vi "ncs_breath.vi"() -> ()   [LabVIEW 2016]
uses:
  <instrlib>/niUSRP/niUSRP Timestamp.ctl
  <instrlib>/niUSRP/niUSRP Write Tx Data (2D CDB).vi
  <instrlib>/niUSRP/niUSRP Fetch Rx Data (2D CDB).vi
  <vilib>/measure/maspectr.llb/FFT Power Spectrum for 1 Chan (CDB).vi
  <vilib>/Analysis/NI_AALBase.lvlib
  <vilib>/Analysis/3filter.llb/Filter Passband Type.ctl
  <vilib>/Analysis/baseanly.llb/IIR Cascade Filter (DBL).vi
  <vilib>/measure/NI_MAPro.lvlib
panel:
  out "Rx Channel tone":dbl
  in  "Preset":string="v1a"
  out "Alarm":bool
  in  "Epsilon":dbl=0.05 format="%#_13g"
  in  "Timer":u16(ring)=90 items=["20min"=1200, "11min"=660, "10min"=600, "5.5min"=330, "2.5min"=150, "1.5min"=90]
  out "Elapsed Time (s)":dbl
  out "Time has Elapsed":bool
  in  "Timer Start":bool
  in  "File Name":string="freq2G_1"
  in  "Path":path=path "D:/Research/SummerFall17Spring18/CnC/NCS/Respiratory/BreathPattern_Cough_Speak/Data"
  out "NCS heartbeat":dbl[](graph)
  in  "Order":dbl=20.0 format="%#_13g"
  in  "High-Cutoff":dbl=8.0 format="%#_13g"
  in  "Low-Cutoff":dbl=0.5 format="%#_13g"
  out "size(s)":i32
  out "Coerced Rx IQ Rate":dbl
  in  "Sampling Rate":i32=500
  out "Gain":dbl=-15.0
  out "Bandwidth":dbl=56000000.0
  out "Coerced Carrier Freq":dbl=2000000000.0 format="%#.17g"
  out "Coerced Tx IQ rate":dbl=1000000.0
  out "error IO":errorcluster={"status"=FALSE, "code"=-1074118647, "source"=""}
  in  "Rx #Samples":i32=20000
  in  "Tab Control 2":enum32{"NI-294x/295x", "NI-2900/2901"}(tab)=enum."NI-2900/2901"
  in  "Rx carrier frequency [Hz]":dbl=2000000000.0 format="%#_6p"
  in  "Tx carrier frequency [Hz]":dbl=1000000000.0 format="%#_6p"
  in  "Start Trigger Time":T1={"whole seconds"=1, "fractional seconds"=0.0}
  in  "Tab Control":T2(tab)
  out "NCS tag Amp":dbl[](graph)=[0.011967714738528729, 0.012021355192189592, 0.012015275039596582, 0.011969166030167903, 0.011958890166168242, 0.012007893820858737, 0.012022893722444085, 0.011978222225113794, 0.011969989939463181, 0.012003099640895068]
  out "NCS tag Phase":dbl[](graph)=[0.011967714738528729, 0.012021355192189592, 0.012015275039596582, 0.011969166030167903, 0.011958890166168242, 0.012007893820858737, 0.012022893722444085, 0.011978222225113794, 0.011969989939463181, 0.012003099640895068]
  out "Tag Amp":dbl[](graph)
  out "Tag Phase":dbl[](graph)
  out "Tx Waveform Graph":waveform(dbl)[](graph)
  out "Baseband Power Spectrum":cluster{"f0":dbl, "df":dbl, "magnitude":dbl[]}[](graph)
  in  "Stop":bool
  in  "Tone Amplitude":dbl=0.707 step=0.05 format="%#.6g"
  in  "Tone Frequency":dbl=10000.0 format="%#_6p"
  in  "Tx Waveform Size":dbl=200.0
  in  "Device Name":refnum<k15>="MyB210"
  in  "Tx Gain":dbl=28.0 format="%#_6f"
  in  "Tx IQ Rate":dbl=1000000.0 format="%#_6p"
  in  "Rx Gain":dbl=32.0 format="%#_6f"
  in  "Rx IQ Rate":dbl=250000.0 format="%#_6p"
  # "Note that on the NI-2900 and NI-2901, both Rx channels share an LO and both Tx channels share an LO. However, on the NI-294x/295x devices, Rx and Tx of channel 0 share an LO and Rx and Tx of channel 1 share an LO."
  # "Rx Settings"
  # "Tx Settings"
  # "Channel 0"
  # "Heartbeat Filter"
  # "This Tx graph should always have end and start tied up since this is being sent in a loop continuously. Otherwise phase jumps will be noticed."
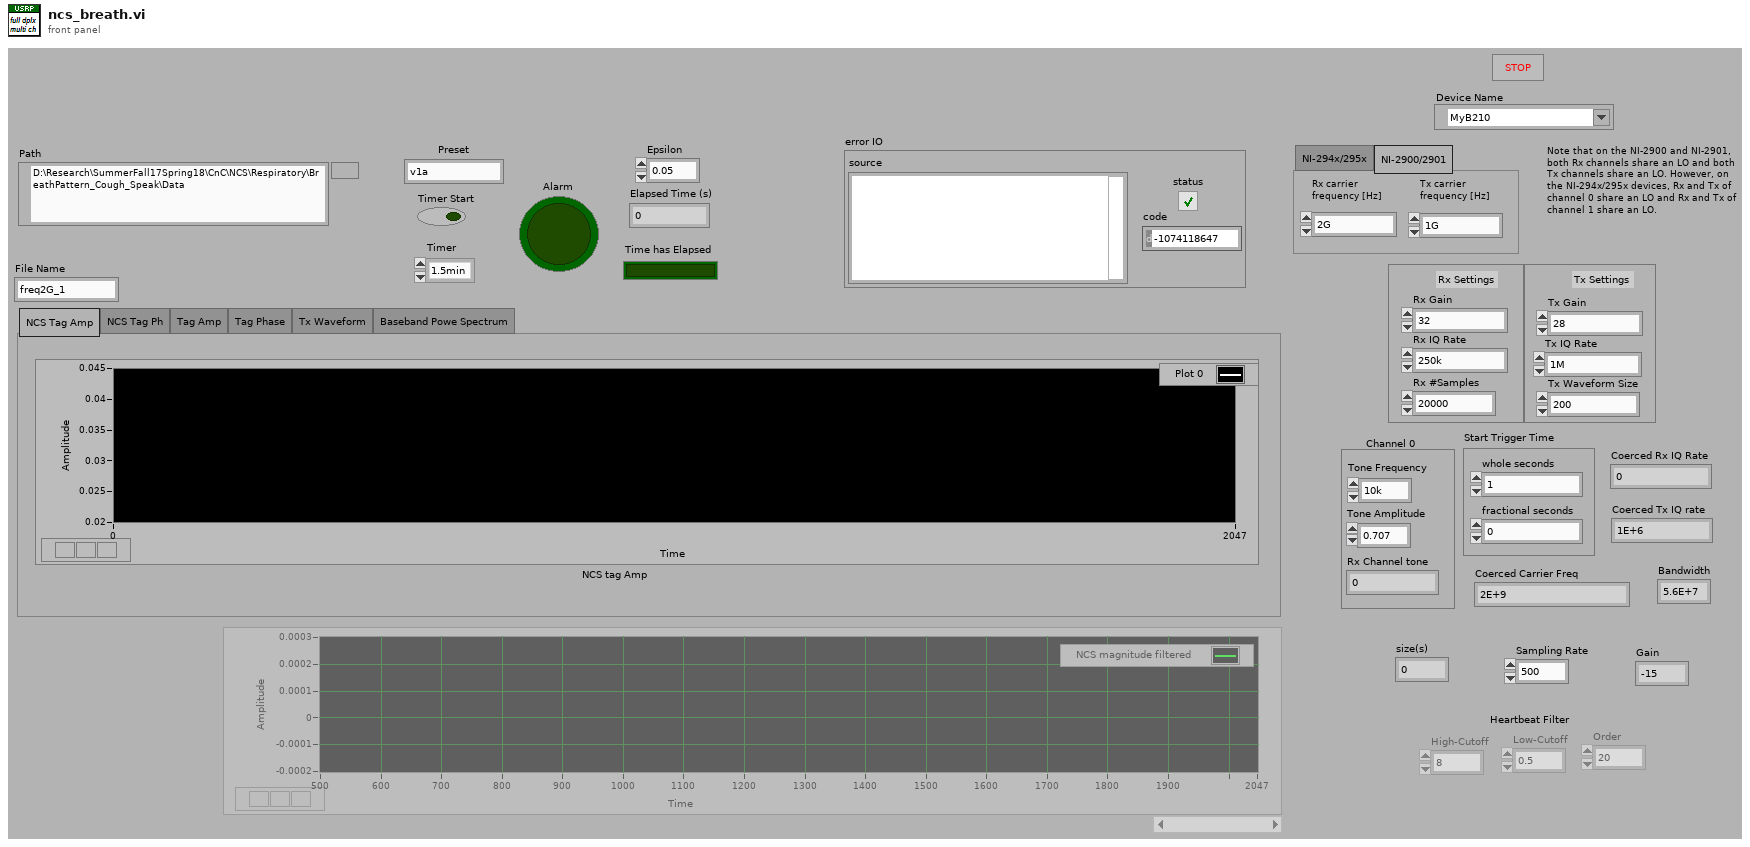
[diagram p1: front panel]
types:
  T1 = typedef "niUSRP Timestamp.ctl" = cluster{"whole seconds":u64, "fractional seconds":dbl}
  T2 = enum32{"NCS Tag Amp", "NCS Tag Ph", "Tag Amp", "Tag Phase", "Tx Waveform", "Baseband Powe Spectrum"}
  T3 = typedef "NI_AALBase.lvlib/Filter Passband Type.ctl" = enum32{"Lowpass", "Highpass", "Bandpass", "Bandstop"}
  T4 = cluster{"filter structure":enum32{"IIR 2nd Order", "IIR 4th Order"}, "Reverse Coefficients":dbl[], "Forward Coefficients":dbl[]}
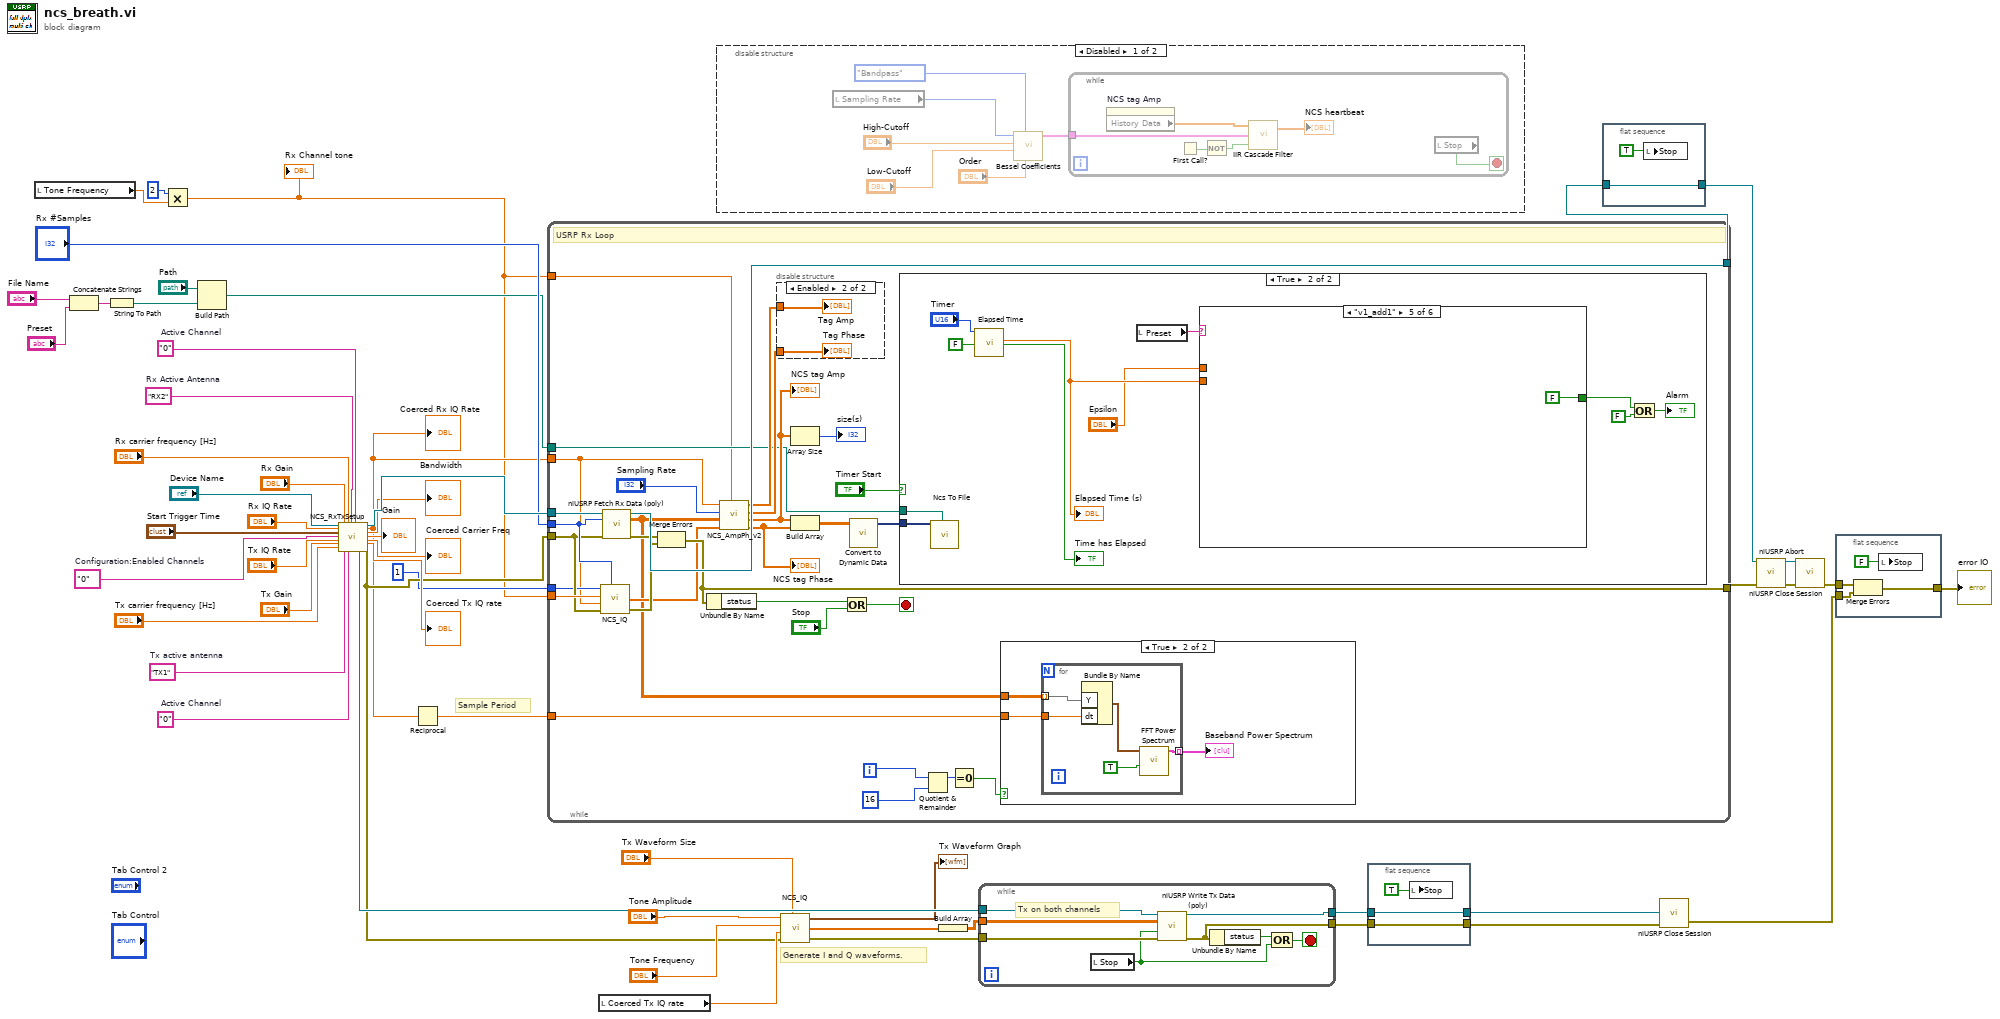
[diagram p0: block diagram]
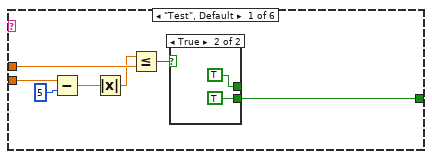
[diagram p5: hidden frame]
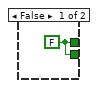
[diagram p6: hidden frame]
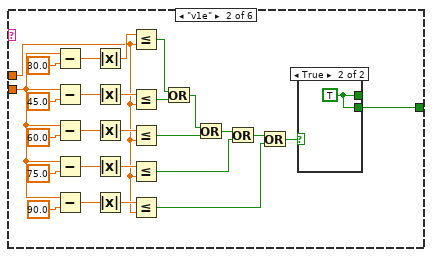
[diagram p7: hidden frame]
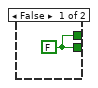
[diagram p8: hidden frame]
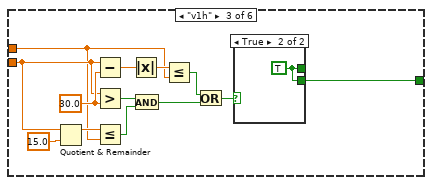
[diagram p9: hidden frame]
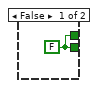
[diagram p10: hidden frame]
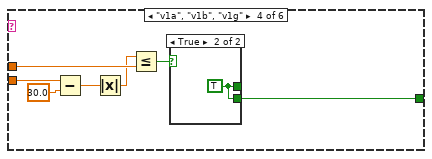
[diagram p11: hidden frame]
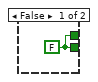
[diagram p12: hidden frame]
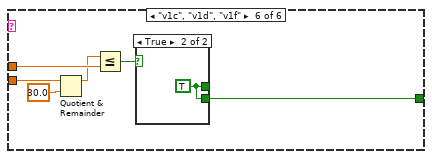
[diagram p13: hidden frame]
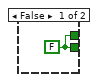
[diagram p14: hidden frame]
diagram:
  w10 = "0"  # Active Channel
  w11 = "0"  # Active Channel
  w45 = "RX2"  # Rx Active Antenna
  w41 = "TX1"  # Tx active antenna
  w27 = "0"  # Configuration:Enabled Channels
  # "Sample Period"
  # "Generate I and Q waveforms."
  n1 = local read "Tone Frequency"() -> (w26:dbl)
  n2 = Concatenate Strings("File Name", "Preset") -> (w5:string)
  n3 = String To Path(string=w5) -> (path=w9:path)
  n4 = Multiply(x=2, y=w26) -> (x*y=w1:dbl)
  "Rx Channel tone" <- w1
  n5 = Build Path(base path="Path", name or relative path=w9) -> (appended path=w7:path)
  n6 = call "NCS_RxTxSetup.vi"("Device Name"="Device Name", "Rx IQ Rate"="Rx IQ Rate", "Start Trigger Time"="Start Trigger Time", "Configuration:Enabled Channels"=w27, "Tx IQ Rate"="Tx IQ Rate", "Tx Gain"="Tx Gain", "Tx carrier frequency [Hz]"="Tx carrier frequency [Hz]", "Rx Gain"="Rx Gain", "Tx active antenna"=w41, "Rx carrier frequency [Hz]"="Rx carrier frequency [Hz]", "Active Channel"=w10, "Rx Active Antenna"=w45, "Active Channel 2"=w11) -> ("Tx session handle out"=w52:refnum<k15>, "Rx Session Handle out"=w53:refnum<k15>, "Coerced Rx IQ Rate"=w3:dbl, "Bandwidth"=→"Bandwidth":dbl, "Gain"=→"Gain":dbl, "Carrier Frequency"=→"Coerced Carrier Freq":dbl, "IQ Rate 2"=→"Coerced Tx IQ rate":dbl, "error out"=w21:errorcluster)  [unwired: 7 in]
  "Coerced Rx IQ Rate" <- w3
  n7 = Reciprocal(x=w3) -> (1/x=w2:dbl)
  n8 = while {
    tunnel: w53 -> [w84]
    tunnel: w21 -> [w76]
    tunnel: [w83] -> w37
    tunnel: "Rx #Samples" -> [w78]
    tunnel: w3 -> [w72]
    tunnel: [w73] -> w29
    tunnel: w1 -> [w77]
    tunnel: 1 -> [w74]
    tunnel: w7 -> [w63]
    tunnel: w2 -> [w57]
    tunnel: w1 -> [w54]
    i -> [w56]
    stop <- w79 stop-if-true
    # "USRP Rx Loop"
    n9 = call "NCS_IQ.vi"("Tone Amplitude"=w74, "Waveform Size"=w78, "Tone Frequency"=w77, "Coerced IQ rate"=w72, "error in (no error)"=w76) -> ("IQ waveform array"=w71:cdb[], "error out"=w75:errorcluster)  [unwired: 1 in, 1 out]
    n10 = call-poly <instrlib>:"niUSRP Fetch Rx Data (poly).vi"("session handle"=w84, "number of samples"=w78, "error in (no error)"=w76) -> ("session handle out"=w83:refnum<k15>, "data"=w58:cdb[][], "error out"=w80:errorcluster)  [unwired: 9 in, 1 out]
    n11 = Merge Errors(w80, w75) -> (w73:errorcluster)
    n12 = Unbundle By Name(w73) -> ("status"=w82:bool)
    n13 = call "NCS_AmpPh_v2.vi"("Rx Channel Tone"=w54, "IQ"=w71, "data"=w58, "Sampling Rate"="Sampling Rate", "Coerced Rx IQ Rate"=w72) -> ("Phase DownSampled"=w64:dbl[], "Amp DownSampled"=w65:dbl[], "Phase"=w70:dbl[], "Amplitude"=w68:dbl[])  [unwired: 3 in]
    "NCS tag Amp" <- w65
    "NCS tag Phase" <- w64
    n14 = disable-structure shown="Enabled" {
      disable-tunnel: w68 -> [_ w177]
      disable-tunnel: w70 -> [_ w176]
      frame Disabled {
      }
      frame Enabled {
        "Tag Amp" <- w177
        "Tag Phase" <- w176
      }
    }
    n15 = Array Size(array=w65) -> (size(s)=→"size(s)":i32)
    n16 = Build Array(w65, w64) -> (w66:dbl[][])
    n17 = Or(x=w82, y="Stop") -> (x .or. y?=w79:bool)
    n18 = call "Convert to Dynamic Data"("2D Array"=w66) -> ("Dynamic Data Type"=w62:dynamicdata)  [unwired: 3 in]
    n19 = case shown="True" "Timer Start" {
      tunnel: w63 -> [_ w103]
      tunnel: w62 -> [_ w102]
      frame False {
      }
      frame True {
        n20 = call "Ncs To File"("Signals"=w102, "Filename"=w103) -> ()  [unwired: 15 in, 3 out]
        n21 = call "Elapsed Time"("Time Target (s)"="Timer", "Auto Reset"=FALSE) -> ("Elapsed Time (s)"=w98:dbl, "Time has Elapsed"=→"Time has Elapsed":bool)  [unwired: 10 in, 6 out]
        "Elapsed Time (s)" <- w98
        n22 = local read "Preset"() -> (w93:string)
        n23 = case shown="\"v1_add1\"" w93 {
          tunnel: w98 -> [w110 w121 w149 w162 _ w171]
          tunnel: "Epsilon" -> [w107 w115 w146 w161 _ w170]
          tunnel: [w106 w129 w152 w163 FALSE w172] -> w95
          frame "Test", Default {
            n24 = Subtract(x=w110, y=5) -> (x-y=w108:dbl)
            n25 = Absolute Value(x=w108) -> (abs(x)=w105:dbl)
            n26 = Less Or Equal?(x=w105, y=w107) -> (x <= y?=w104:bool)
            n27 = case shown="True" w104 {
              tunnel: [w111 TRUE] -> w106
              tunnel: [w111 TRUE] -> _
              frame False {
                w111 = FALSE
              }
              frame True {
              }
            }
          }
          frame "v1e" {
            n28 = Subtract(x=w121, y=30.0) -> (x-y=w139:dbl)
            n29 = Subtract(x=w121, y=45.0) -> (x-y=w136:dbl)
            n30 = Subtract(x=w121, y=60.0) -> (x-y=w132:dbl)
            n31 = Subtract(x=w121, y=75.0) -> (x-y=w128:dbl)
            n32 = Subtract(x=w121, y=90.0) -> (x-y=w124:dbl)
            n33 = Absolute Value(x=w139) -> (abs(x)=w138:dbl)
            n34 = Absolute Value(x=w136) -> (abs(x)=w135:dbl)
            n35 = Absolute Value(x=w132) -> (abs(x)=w131:dbl)
            n36 = Absolute Value(x=w128) -> (abs(x)=w127:dbl)
            n37 = Absolute Value(x=w124) -> (abs(x)=w123:dbl)
            n38 = Less Or Equal?(x=w138, y=w115) -> (x <= y?=w137:bool)
            n39 = Less Or Equal?(x=w135, y=w115) -> (x <= y?=w133:bool)
            n40 = Less Or Equal?(x=w131, y=w115) -> (x <= y?=w120:bool)
            n41 = Less Or Equal?(x=w127, y=w115) -> (x <= y?=w118:bool)
            n42 = Less Or Equal?(x=w123, y=w115) -> (x <= y?=w116:bool)
            n43 = Or(x=w137, y=w133) -> (x .or. y?=w125:bool)
            n44 = Or(x=w125, y=w120) -> (x .or. y?=w119:bool)
            n45 = Or(x=w119, y=w118) -> (x .or. y?=w117:bool)
            n46 = Or(x=w117, y=w116) -> (x .or. y?=w114:bool)
            n47 = case shown="True" w114 {
              tunnel: [w141 w142] -> _
              tunnel: [w141 w142] -> w129
              frame False {
                w141 = FALSE
              }
              frame True {
                w142 = TRUE
              }
            }
          }
          frame "v1h" {
            w151 = 30.0 ("y")
            n48 = Quotient & Remainder(x=w149, y=15.0) -> (x-y*floor(x/y)=w147:dbl)  [unwired: 1 out]
            n49 = Subtract(x=w149, y=w151) -> (x-y=w155:dbl)
            n50 = Greater?(x=w149, y=w151) -> (0:w150:bool)
            n51 = Less Or Equal?(x=w147, y=w146) -> (x <= y?=w145:bool)
            n52 = Absolute Value(x=w155) -> (abs(x)=w154:dbl)
            n53 = And(x=w150, y=w145) -> (x .and. y?=w144:bool)
            n54 = Less Or Equal?(x=w154, y=w146) -> (x <= y?=w153:bool)
            n55 = Or(x=w153, y=w144) -> (x .or. y?=w143:bool)
            n56 = case shown="True" w143 {
              tunnel: [w156 w157] -> _
              tunnel: [w156 w157] -> w152
              frame False {
                w156 = FALSE
              }
              frame True {
                w157 = TRUE
              }
            }
          }
          frame "v1a", "v1b", "v1g" {
            n57 = Subtract(x=w162, y=30.0) -> (x-y=w159:dbl)
            n58 = Absolute Value(x=w159) -> (abs(x)=w158:dbl)
            n59 = Less Or Equal?(x=w158, y=w161) -> (x <= y?=w160:bool)
            n60 = case shown="True" w160 {
              tunnel: [w165 w166] -> _
              tunnel: [w165 w166] -> w163
              frame False {
                w165 = FALSE
              }
              frame True {
                w166 = TRUE
              }
            }
          }
          frame "v1_add1" {
          }
          frame "v1c", "v1d", "v1f" {
            n61 = Quotient & Remainder(x=w171, y=30.0) -> (x-y*floor(x/y)=w168:dbl)  [unwired: 1 out]
            n62 = Less Or Equal?(x=w168, y=w170) -> (x <= y?=w169:bool)
            n63 = case shown="True" w169 {
              tunnel: [w174 w175] -> _
              tunnel: [w174 w175] -> w172
              frame False {
                w174 = FALSE
              }
              frame True {
                w175 = TRUE
              }
            }
          }
        }
        n64 = Or(x=w95, y=FALSE) -> (x .or. y?=→"Alarm":bool)
      }
    }
    n65 = Quotient & Remainder(x=w56, y=16) -> (x-y*floor(x/y)=w60:i32)  [unwired: 1 out]
    n66 = Equal To 0?(x=w60) -> (x = 0?=w59:bool)
    n67 = case shown="True" w59 {
      tunnel: w58 -> [_ w87]
      tunnel: w57 -> [_ w86]
      frame False {
      }
      frame True {
        n68 = for {
          tunnel: w87 -> [w90] mode=indexing
          tunnel: w86 -> [w89]
          tunnel: [w88] -> w85 mode=indexing
          n69 = Bundle By Name("Y"=w90, "dt"=w89) -> (w91:waveform(cdb))  [unwired: 1 in]
          n70 = call-poly <vilib>:"FFT Power Spectrum.vi"("dB On (F)"=TRUE, "time signal"=w91) -> ("power spectrum"=w88:cluster{"f0":dbl, "df":dbl, "magnitude":dbl[]})  [unwired: 6 in, 3 out]
        }
        "Baseband Power Spectrum" <- w85
      }
    }
  }
  n71 = local read "Coerced Tx IQ rate"() -> (w22:dbl)
  n72 = disable-structure shown="Disabled" {
    frame Disabled {
      n73 = local read "Sampling Rate"() -> (w182:i32)
      n74 = call <vilib>:"Bessel Coefficients.vi"("order"="Order", "filter type"=Filter_Passband_Type."Bandpass", "low cutoff freq: fl"="Low-Cutoff", "high cutoff freq: fh"="High-Cutoff", "sampling freq: fs"=w182) -> ("IIR Filter Cluster"=w178:T4)  [unwired: 5 in, 1 out]
      n75 = while {
        tunnel: w178 -> [w186]
        stop <- w188 stop-if-true
        n76 = property on="NCS tag Amp" class="WaveformChart (strict)"() -> ("History Data"=w187:dbl[])  [unwired: 2 in, 2 out]
        n77 = First Call?() -> (First Call?: T/F=w189:bool)
        n78 = Not(x=w189) -> (.not. x?=w185:bool)
        n79 = call-poly <vilib>:"IIR Cascade Filter.vi"("init/cont (init:F)"=w185, "IIR Filter Cluster"=w186, "X"=w187) -> ("Filtered X"=→"NCS heartbeat":dbl[])  [unwired: 1 out]
        n80 = local read "Stop"() -> (w188:bool)
      }
    }
    frame Enabled {
    }
  }
  n81 = call "NCS_IQ.vi"("Tone Amplitude"="Tone Amplitude", "Waveform Size"="Tx Waveform Size", "Tone Frequency"="Tone Frequency", "Coerced IQ rate"=w22, "error in (no error)"=w21) -> ("IQ waveform"=→"Tx Waveform Graph":waveform(dbl)[], "IQ waveform array"=w19:cdb[], "error out"=w20:errorcluster)  [unwired: 1 in]
  n82 = Build Array(w19) -> (w49:cdb[][])
  n83 = while {
    tunnel: w52 -> [w197]
    tunnel: w20 -> [w196]
    tunnel: [w194] -> w40
    tunnel: [w192] -> w35
    tunnel: w49 -> [w190]
    stop <- w193 stop-if-true
    # "Tx on both channels"
    n84 = local read "Stop"() -> (w191:bool)
    n85 = call-poly <instrlib>:"niUSRP Write Tx Data (poly).vi"("session handle"=w197, "data"=w190, "end of data?"=w191, "error in (no error)"=w196) -> ("session handle out"=w192:refnum<k15>, "error out"=w194:errorcluster)  [unwired: 10 in]
    n86 = Unbundle By Name(w194) -> ("status"=w195:bool)
    n87 = Compound Arithmetic op=OR(w195, w191) -> (w193:bool)
  }
  n88 = flat-sequence {
    tunnel: [w199] -> w39
    tunnel: w40 -> [w199]
    tunnel: [w198] -> w36
    tunnel: w35 -> [w198]
    frame #0 {
      n89 = local write "Stop"(TRUE ("STOP")) -> ()
    }
  }
  n90 = flat-sequence {
    tunnel: [w201] -> w38
    tunnel: w37 -> [w201]
    frame #0 {
      n91 = local write "Stop"(TRUE ("STOP")) -> ()
    }
  }
  n92 = call <instrlib>:"niUSRP Close Session.vi"("session handle"=w36, "error in (no error)"=w39) -> ("error out"=w34:errorcluster)  [unwired: 13 in]
  n93 = call <instrlib>:"niUSRP Abort.vi"("session handle"=w38, "error in (no error)"=w29) -> ("session handle out"=w51:refnum<k15>, "error out"=w50:errorcluster)  [unwired: 12 in]
  n94 = call <instrlib>:"niUSRP Close Session.vi"("session handle"=w51, "error in (no error)"=w50) -> ("error out"=w31:errorcluster)  [unwired: 13 in]
  n95 = flat-sequence {
    tunnel: w34 -> [w205]
    tunnel: [w204] -> w32
    tunnel: w31 -> [w203]
    frame #0 {
      n96 = Merge Errors(w203, w205) -> (w204:errorcluster)
      n97 = local write "Stop"(FALSE ("STOP")) -> ()
    }
  }
  "error IO" <- w32
